vi "Periodic Tasks.vi"(8 "error in":errorcluster) -> ()   [LabVIEW 2019]
doc: "This VI runs in parallel to other tasks. It can contain as many user-defined periodic loops as you need. These can carry out PID or other sorts of timed response."
uses:
  2019-Robot-Code/Swerve Drive/Vision Data.ctl
  <vilib>/Rock Robotics/Network Tables/NT Read Number.vi
  Robot Global Data.vi
  <vilib>/Rock Robotics/WPI/ThirdParty/Phoenix-LabVIEW/Motor Controller/Get/CTRE_Phoenix_MotorController_IntegratedSensorData_TalonFX.vi
  <vilib>/Rock Robotics/Network Tables/NT Write Variant.vi
  <vilib>/Rock Robotics/Network Tables/NT Write Number.vi
  <vilib>/numeric/Random Number (Range) U64.vi
panel:
  out "Position":dbl format="%.2f"
  out "Distance":dbl
  out "Value 4":i16
  out "Value 3":i16
  out "Value 2":i16
  out "Value":i16
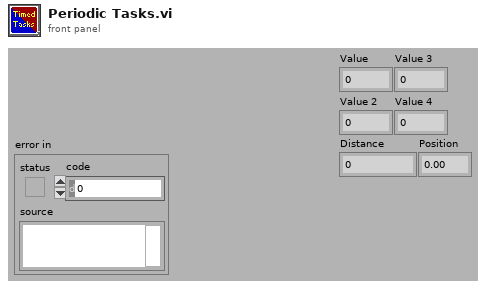
[diagram p1: front panel]
types:
  T1 = typedef "Vision Data.ctl" = cluster{"xOffset":dbl, "yOffset":dbl, "area":dbl, "skewOffset":dbl, "hasTarget":dbl}
  T2 = cluster{"Yaw":dbl, "Roll":dbl, "Pitch":dbl, "Heading":dbl, "Fused Heading":dbl}
  T3 = typedef "WPI_AnalogChannelDevRef.ctl" = cluster{"DevStatus":errorcluster, "Analog Channel":T4}
  T4 = typedef "FPGA_AIChannel.ctl" = enum8{"AI 0", "AI 1", "AI 2", "AI 3", "AI MXP 0", "AI MXP 1", "AI MXP 2", "AI MXP 3", "Invalid"}
  T5 = typedef "WPI_MotorControlDeviceRef.ctl" = cluster{"DeviceStatus":errorcluster, "Type":T6, "PWM":cluster{"PWM Channel":T7, "DeadBand":T8}, "CAN":cluster{"Device Number":u8, "SetOutput VI Ref":variant, "GetOutput VI Ref":variant, "Enable VI Ref":variant, "Disable VI Ref":variant, "Data":variant}, "Invert":bool, "DIO PWM":cluster{"PWM \"Enable\" Channel":T7, "DIOChannel":T9, "PWM Rate":dbl}}
  T6 = typedef "WPI_MotorControlType.ctl" = enum16{"PWM", "CAN", "DIO PWM"}
  T7 = typedef "FPGA_DIOPWMChannel.ctl" = enum8{"PWM 0", "PWM 1", "PWM 2", "PWM 3", "PWM 4", "PWM 5", "PWM 6", "PWM 7", "PWM 8", "PWM 9", "PWM MXP 0", "PWM MXP 1", "PWM MXP 2", "PWM MXP 3", "PWM MXP 4", "PWM MXP 5", "PWM MXP 6", "PWM MXP 7", "PWM MXP 8", "PWM MXP 9", "Invalid"}
  T8 = typedef "WPI_PWMDeadband.ctl" = cluster{"Name":string, "maxPositivePwm":i32, "minPositivePwm":i32, "centerPwm":i32, "maxNegativePwm":i32, "minNegativePwm":i32, "angularRange":u16}
  T9 = typedef "FPGA_DIOChannel.ctl" = enum8{"DIO 0", "DIO 1", "DIO 2", "DIO 3", "DIO 4", "DIO 5", "DIO 6", "DIO 7", "DIO 8", "DIO 9", "DIO MXP 0", "DIO MXP 1", "DIO MXP 2", "DIO MXP 3", "DIO MXP 4", "DIO MXP 5", "DIO MXP 6", "DIO MXP 7", "DIO MXP 8", "DIO MXP 9", "DIO MXP 10", "DIO MXP 11", "DIO MXP 12", "DIO MXP 13", "DIO MXP 14", "DIO MXP 15", "SPI Port CS1", "SPI Port CS2", "SPI Port CS3", "SPI Port MISO", "SPI Port MOSI", "Invalid"}
  T10 = typedef "WPI_EncoderDevRef.ctl" = cluster{"DevStatus":errorcluster, "EncoderIndex":T11, "CounterIndex":T12, "DistancePerCount":dbl, "Decoding Type":T13}
  T11 = typedef "FPGA_EncoderIdx.ctl" = enum8{"Enc 0", "Enc 1", "Enc 2", "Enc 3", "Enc 4", "Enc 5", "Enc 6", "Enc 7", "Invalid"}
  T12 = typedef "FPGA_CounterCtrSystemIndex.ctl" = enum8{"Ctr 0", "Ctr 1", "Ctr 2", "Ctr 3", "Ctr 4", "Ctr 5", "Ctr 6", "Ctr 7", "Invalid"}
  T13 = typedef "WPI_EncoderType.ctl" = enum16{"1x", "2x", "4x"}
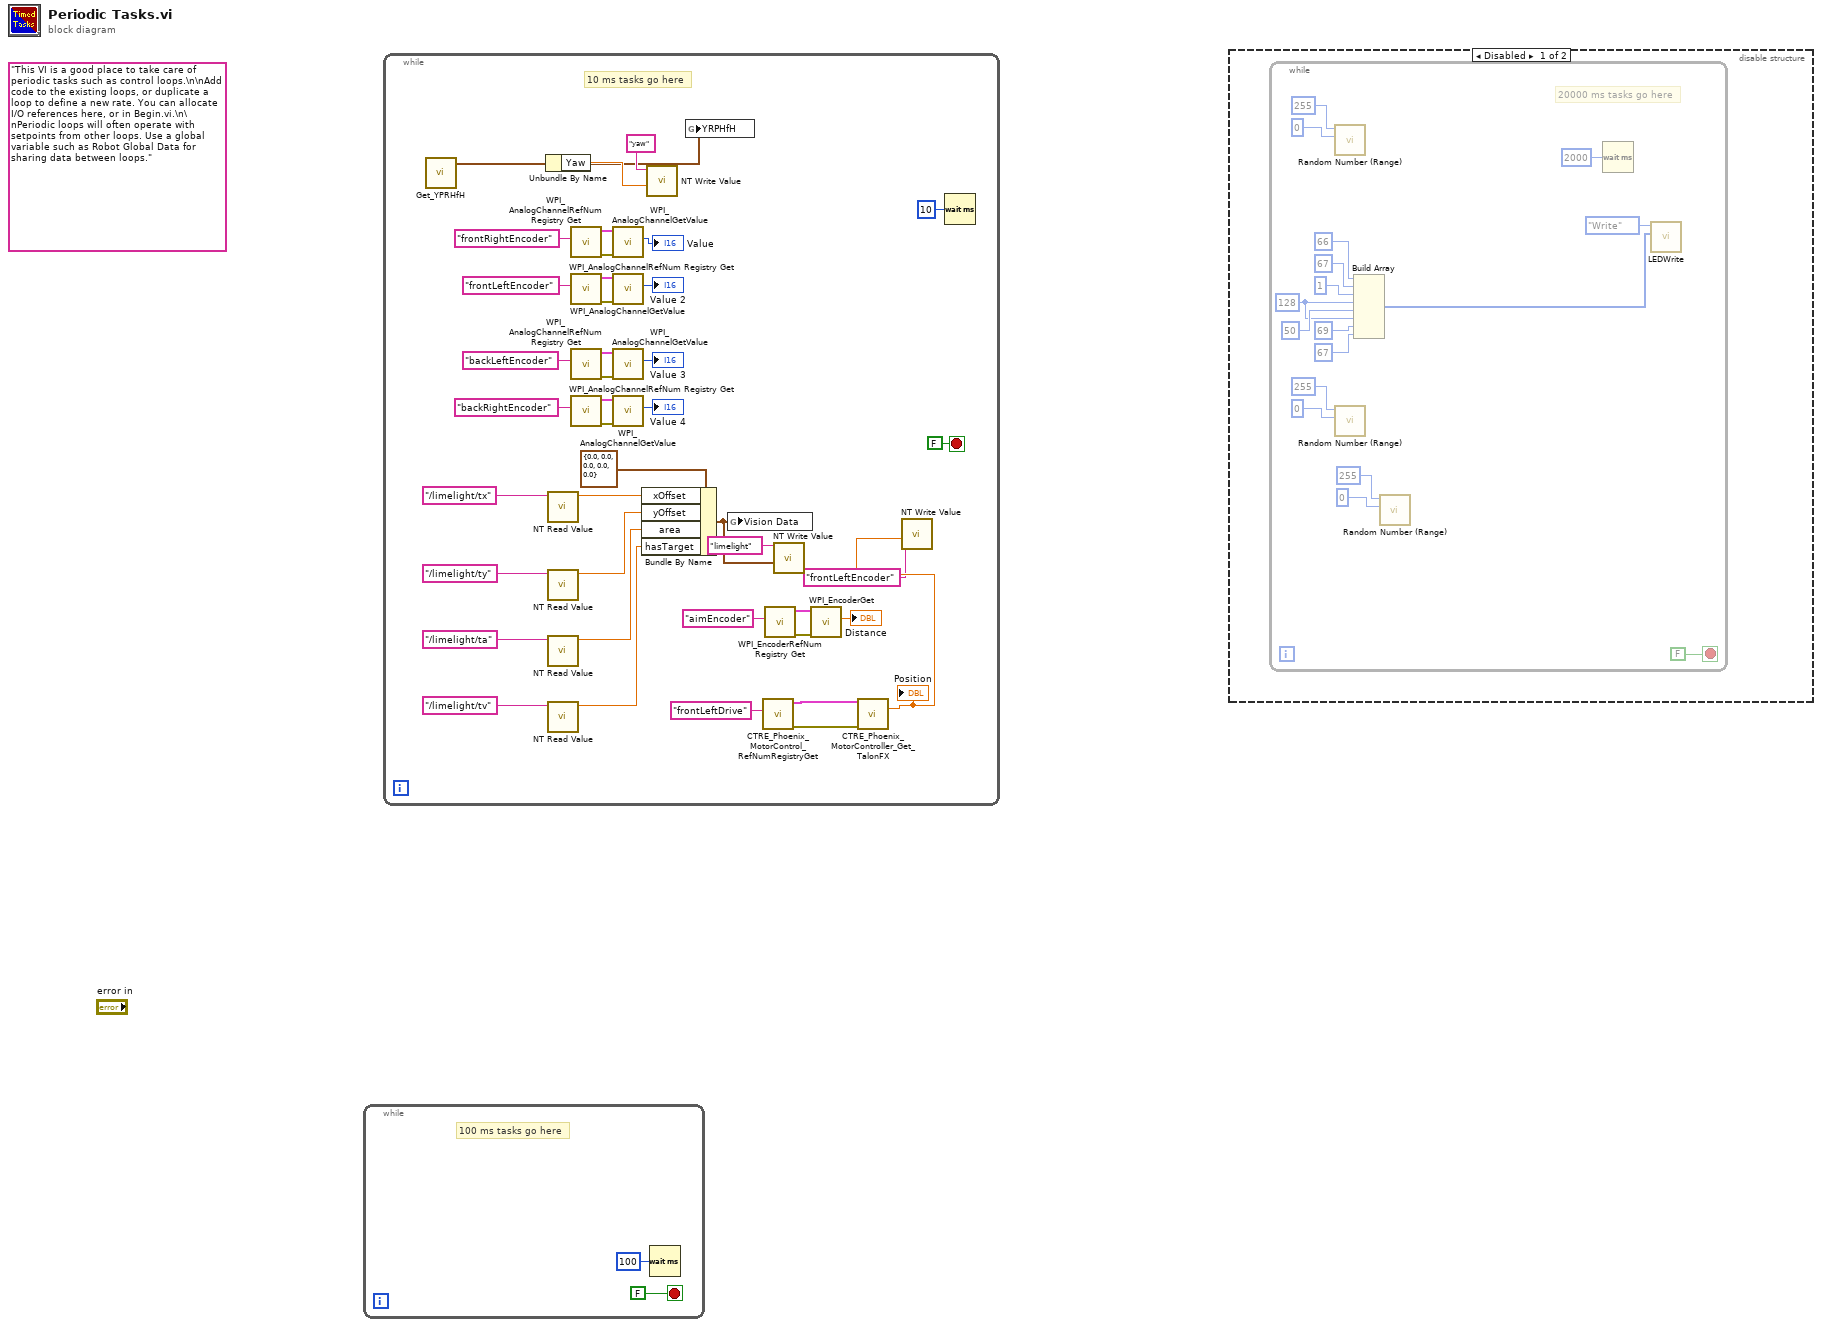
[diagram p0: block diagram]
diagram:
  (unwired) "This VI is a good place to take care of periodic tasks such as control loops.\n\nAdd code to the existing loops, or duplicate a loop to define a new rate. You can allocate I/O references here, or in Begin.vi.\n\nPeriodic loops will often operate with setpoints from other loops. Use a global variable such as Robot Global Data for sharing data between loops."
  n1 = while {
    stop <- FALSE stop-if-true
    # "100 ms tasks go here"
    n2 = Wait (ms)(milliseconds to wait=u32 100) -> ()  [unwired: 1 out]
  }
  n3 = while {
    stop <- FALSE stop-if-true
    # "10 ms tasks go here"
    n4 = call <vilib>:"Get_YPRHfH.vi"() -> ("YRPHfH"=w39:T2)  [unwired: 11 in]
    n5 = Unbundle By Name(w39) -> ("Yaw"=w41:dbl)
    n6 = call-poly <vilib>:"NT Read Value.vi"("Name"="/limelight/tx") -> ("Numeric"=w16:dbl)  [unwired: 9 in, 1 out]
    n7 = call-poly <vilib>:"NT Read Value.vi"("Name"="/limelight/ty") -> ("Numeric"=w17:dbl)  [unwired: 9 in, 1 out]
    n8 = call-poly <vilib>:"NT Read Value.vi"("Name"="/limelight/ta") -> ("Numeric"=w18:dbl)  [unwired: 9 in, 1 out]
    n9 = call-poly <vilib>:"NT Read Value.vi"("Name"="/limelight/tv") -> ("Numeric"=w14:dbl)  [unwired: 9 in, 1 out]
    n10 = call <vilib>:"WPI_AnalogChannelRefNum Registry Get.vi"("refnum name"="frontRightEncoder") -> ("error out"=w34:errorcluster, "AIDeviceRef"=w33:T3)  [unwired: 9 in]
    n11 = call <vilib>:"WPI_AnalogChannelRefNum Registry Get.vi"("refnum name"="frontLeftEncoder") -> ("error out"=w28:errorcluster, "AIDeviceRef"=w27:T3)  [unwired: 9 in]
    n12 = call <vilib>:"WPI_AnalogChannelRefNum Registry Get.vi"("refnum name"="backLeftEncoder") -> ("error out"=w36:errorcluster, "AIDeviceRef"=w35:T3)  [unwired: 9 in]
    n13 = call <vilib>:"WPI_AnalogChannelRefNum Registry Get.vi"("refnum name"="backRightEncoder") -> ("error out"=w38:errorcluster, "AIDeviceRef"=w37:T3)  [unwired: 9 in]
    n14 = call <vilib>:"WPI_AnalogChannelGetValue.vi"("error in (no error)"=w34, "AIDeviceRef"=w33) -> ("Value"=→"Value":i16)  [unwired: 7 in, 2 out]
    n15 = call <vilib>:"WPI_AnalogChannelGetValue.vi"("error in (no error)"=w28, "AIDeviceRef"=w27) -> ("Value"=→"Value 2":i16)  [unwired: 7 in, 2 out]
    n16 = call <vilib>:"WPI_AnalogChannelGetValue.vi"("error in (no error)"=w36, "AIDeviceRef"=w35) -> ("Value"=→"Value 3":i16)  [unwired: 7 in, 2 out]
    n17 = call <vilib>:"WPI_AnalogChannelGetValue.vi"("error in (no error)"=w38, "AIDeviceRef"=w37) -> ("Value"=→"Value 4":i16)  [unwired: 7 in, 2 out]
    n18 = Bundle By Name(cluster=T1 {"xOffset"=0.0, "yOffset"=0.0, "area"=0.0, "skewOffset"=0.0, "hasTarget"=0.0} ("Vision Data"), "xOffset"=w16, "yOffset"=w17, "area"=w18, "hasTarget"=w14) -> (w6:T1)
    n19 = call-poly <vilib>:"NT Write Value.vi"("Numeric"=w41, "Name"="yaw") -> ()  [unwired: 9 in, 1 out]
    n20 = global write "Robot Global Data.vi" "YRPHfH"(w39) -> ()
    n21 = global write "Robot Global Data.vi" "Vision Data"(w6) -> ()
    n22 = call <vilib>:"CTRE_Phoenix_MotorControl_RefNumRegistryGet.vi"("refnum name"="frontLeftDrive") -> ("error out"=w9:errorcluster, "PhoenixMotorControlDevRef"=w7:T5)  [unwired: 9 in]
    n23 = call <vilib>:"WPI_EncoderRefNum Registry Get.vi"("refnum name"="aimEncoder") -> ("error out"=w13:errorcluster, "EncoderDevRef"=w12:T10)  [unwired: 9 in]
    n24 = call-poly <vilib>:"NT Write Value.vi"("Variant"=w6, "Name"="limelight") -> ()  [unwired: 9 in, 1 out]
    n25 = call <vilib>:"WPI_EncoderGet.vi"("error in (no error)"=w13, "EncoderDevRef"=w12) -> ("Distance"=→"Distance":dbl)  [unwired: 4 in, 5 out]
    n26 = call-poly <vilib>:"CTRE_Phoenix_MotorController_Get_TalonFX.vi"("PhoenixMotorControlDevRef"=w7, "error in"=w9) -> ("Position"=w4:dbl)  [unwired: 9 in, 4 out]
    "Position" <- w4
    n27 = call-poly <vilib>:"NT Write Value.vi"("Numeric"=w4, "Name"="frontLeftEncoder") -> ()  [unwired: 9 in, 1 out]
    n28 = Wait (ms)(milliseconds to wait=u32 10) -> ()  [unwired: 1 out]
  }
  n29 = disable-structure shown="Disabled" {
    frame Disabled {
      n30 = while {
        stop <- FALSE stop-if-true
        w46 = u64 128 ("element")
        # "20000 ms tasks go here"
        n31 = call-poly <vilib>:"Random Number (Range).vi"("lower bound (0)"=u64 0, "upper bound (100)"=u64 255) -> ()  [unwired: 9 in, 1 out]
        n32 = call-poly <vilib>:"Random Number (Range).vi"("lower bound (0)"=u64 0, "upper bound (100)"=u64 255) -> ()  [unwired: 9 in, 1 out]
        n33 = Build Array(u64 66 ("element"), u64 67 ("element"), u64 1 ("element"), w46, u64 50 ("element"), w46, u64 69 ("element"), u64 67 ("element")) -> (w48:u64[])
        n34 = call-poly <vilib>:"Random Number (Range).vi"("lower bound (0)"=u64 0, "upper bound (100)"=u64 255) -> ()  [unwired: 9 in, 1 out]
        n35 = Wait (ms)(milliseconds to wait=u32 2000) -> ()  [unwired: 1 out]
        n36 = call "LEDWrite.vi"("Data To Send"=w48, "Enum"=enum16{"Write", "Open"}."Write") -> ()  [unwired: 10 in]
      }
    }
    frame Enabled {
    }
  }
